vi "TestCOMxsquare2.vi"() -> ()   [LabVIEW 2012]
panel:
  in  "xsquare.IClass1":refnum<k7>
  out "数组":dbl[](array[numeric])
  out "x+y":dbl
  in  "数值":dbl
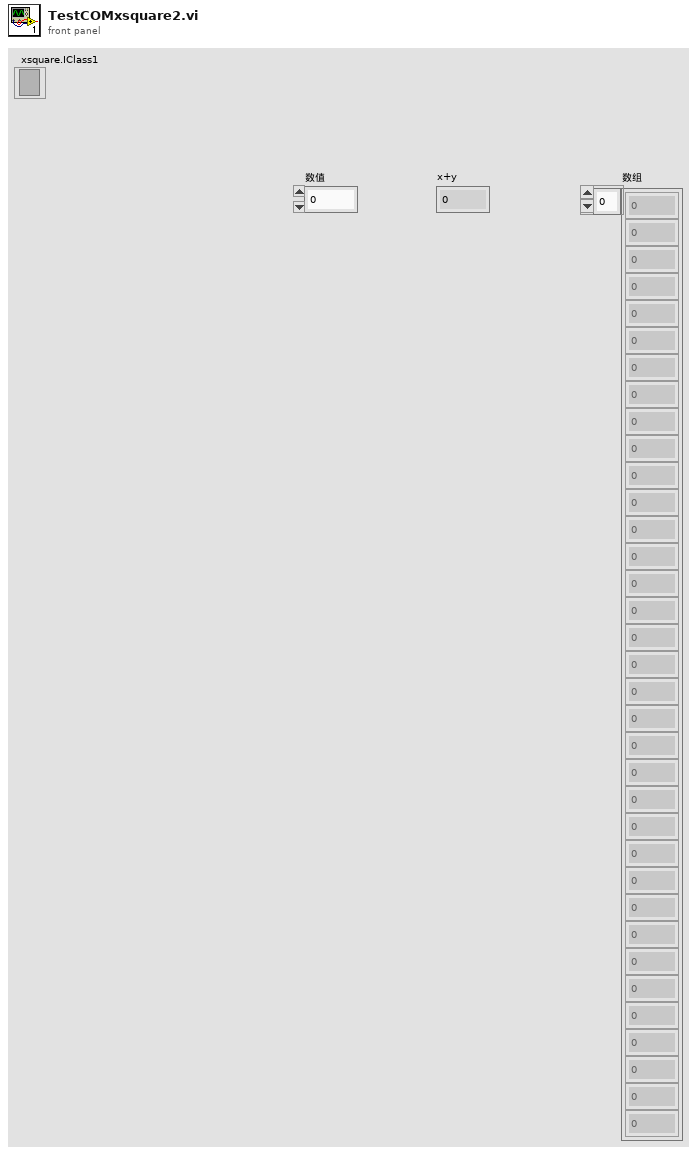
[diagram p1: front panel]
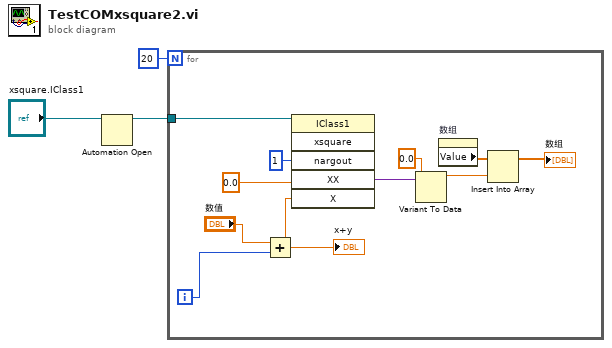
[diagram p0: block diagram]
diagram:
  n1 = Automation Open(Automation Refnum="xsquare.IClass1") -> (Automation Refnum=w3:refnum<k7>)  [unwired: 3 in, 1 out]
  n2 = for {
    N: 20 -> [_]
    tunnel: w3 -> [w14]
    i -> [w8]
    n3 = Add(x="数值", y=w8) -> (x+y=w7:dbl)
    "x+y" <- w7
    n4 = invoke class="IClass1" method="xsquare"(reference=w14, "nargout"=1, "XX"=0.0, "X"=w7) -> ("XX"=w11:variant)  [unwired: 2 in, 5 out]
    n5 = Variant To Data(type=0.0, Variant=w11) -> (data=w6:dbl)  [unwired: 1 in, 1 out]
    n6 = property on="数组" class="Arr (严格)"() -> ("Value"=w4:dbl[])  [unwired: 2 in, 2 out]
    n7 = Insert Into Array(array=w4, new element=w6) -> (→"数组":dbl[])  [unwired: 1 in]
  }
